vi "table_creation.vi"(8 "column information":T1[](array[typedef]), 9 "table_name":string, 11 "connection information":path) -> (0 "error out":errorcluster)   [LabVIEW 2019]
uses:
  <vilib>/addons/database/Auxilliary.llb/DB Tools Column Info.ctl
  <vilib>/addons/database/Auxilliary.llb/DB Tools DataTypes.ctl
  <vilib>/addons/database/Connection.llb/DB Tools Open Connec (Path).vi
  <vilib>/addons/database/NI_Database_API.lvlib
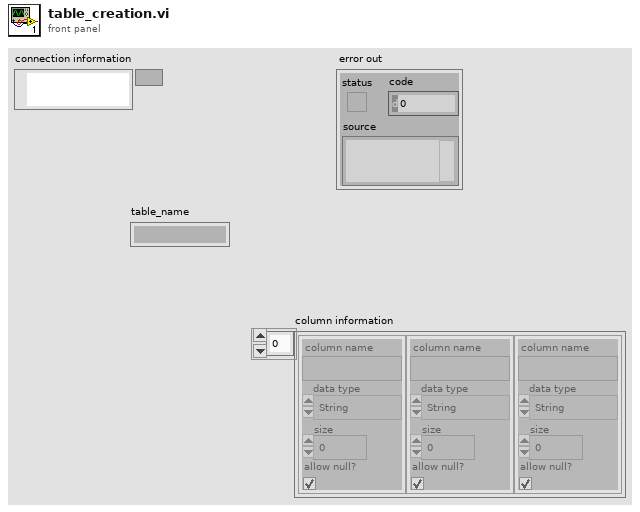
[diagram p1: front panel]
types:
  T1 = typedef "NI_Database_API.lvlib/DB Tools Column Info.ctl" = cluster{"column name":string, "data type":T2, "size":i32, "allow null?":bool}
  T2 = typedef "NI_Database_API.lvlib/DB Tools DataTypes.ctl" = enum16{"String", "Long (I32)", "Single (SGL)", "Double (DBL)", "Date/Time", "Binary"}
  T3 = typedef "NI_Database_API.lvlib/Conn ObjectReference.ctl" = refnum<k1>
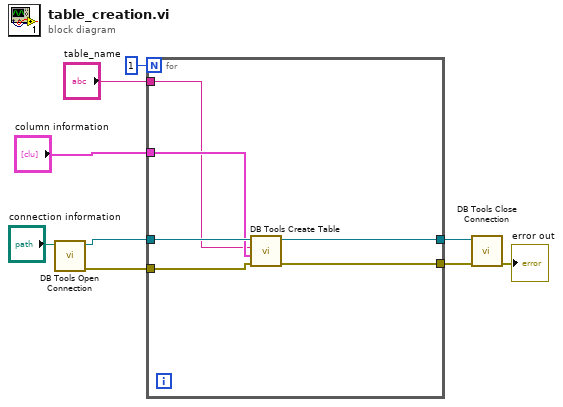
[diagram p0: block diagram]
diagram:
  n1 = call-poly <vilib>:"DB Tools Open Connection.vi"("connection information"="connection information") -> ("error out"=w6:errorcluster, "connection reference"=w9:T3)  [unwired: 7 in]
  n2 = for {
    N: 1 -> [_]
    tunnel: w9 -> [w15]
    tunnel: [w14] -> w8
    tunnel: [w13] -> w7
    tunnel: w6 -> [w12]
    tunnel: "column information" -> [w11]
    tunnel: "table_name" -> [w10]
    n3 = call <vilib>:"DB Tools Create Table.vi"("error in (no error)"=w12, "column information"=w11, "table"=w10, "connection reference"=w15) -> ("error out"=w13:errorcluster, "connection reference out"=w14:T3)  [unwired: 4 in]
  }
  n4 = call <vilib>:"DB Tools Close Connection.vi"("error in (no error)"=w7, "connection reference"=w8) -> ("error out"=→"error out":errorcluster)  [unwired: 5 in]
